vi "Save Image.vi"() -> ()   [LabVIEW 2013]
doc: "This VI imlements the framework and scheduler for your robotics program. It should not be necessary to modify the framework. You are expected to add your code to the VIs called from Robot Main, the ones located in the Team Code within the project."
panel:
  in  "Filename":string="Example.jpg"
  in  "Directory to save images":path=path "c:/images"
  out "Camera error":errorcluster
  out "File error":errorcluster
  out "Image":T1(plugin-control)
  in  "stop":bool
  in  "Save Image":bool
  # "This can be set\nwhile running."
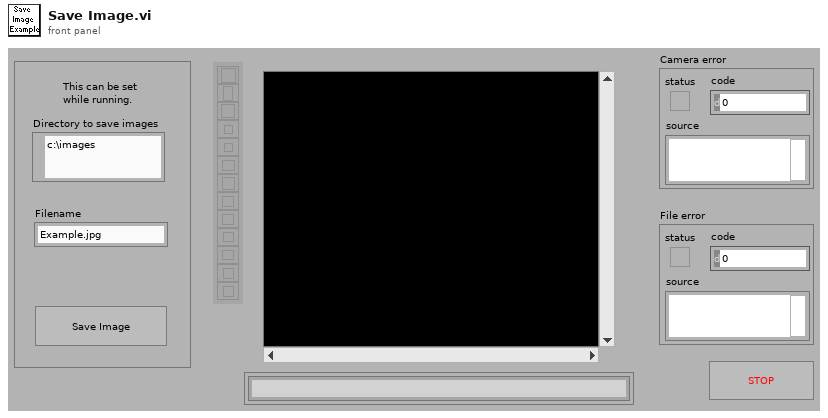
[diagram p1: front panel]
types:
  T1 = typedef "IMAQ Image.ctl" = refnum<image>
  T2 = typedef "Image Type" = u32
  T3 = typedef "WPI_CameraDevRef.ctl" = cluster{"Camera Address":string, "CameraStatus":errorcluster, "Acquire Image Notifier":refnum<notifier>}
  T4 = enum16{"open", "replace", "create", "open or create", "replace or create", "replace or create with confirmation"}
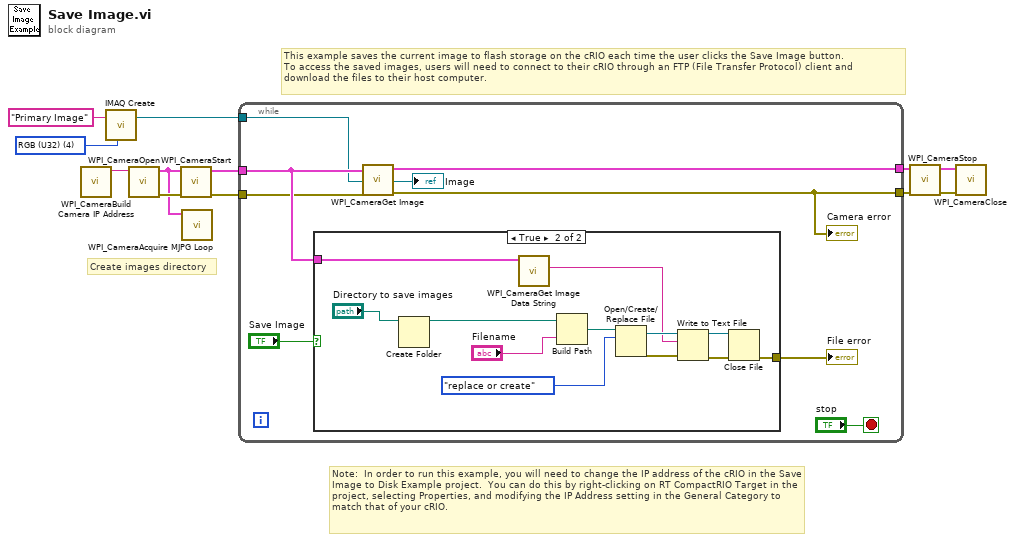
[diagram p0: block diagram]
diagram:
  w5 = T2 4 items=["Grayscale (U8)", "Grayscale (I16)", "Grayscale (SGL)", "Complex (CSG)", "RGB (U32)", "HSL (U32)", "RGB (U64)"] ("Image Type")
  # "Note:  In order to run this example, you will need to change the IP address of the cRIO in the Save Image to Disk Example project.  You can do this by right-clicking on RT CompactRIO Target in the project, selecting Properties, and modifying the IP Address setting in the General Category to match that of your cRIO."
  # "This example saves the current image to flash storage on the cRIO each time the user clicks the Save Image button.\nTo access the saved images, users will need to connect to their cRIO through an FTP (File Transfer Protocol) client and\ndownload the files to their host computer."
  # "Create images directory"
  n1 = call <vilib>:"WPI_CameraBuild Camera IP Address.vi"() -> ("Camera Address"=w1:string)  [unwired: 11 in]
  n2 = call "IMAQ Create"("Image Name"="Primary Image", "Image Type"=w5) -> ("New Image"=w3:T1)  [unwired: 2 in, 2 out]
  n3 = call <vilib>:"WPI_CameraOpen.vi"("Camera Address"=w1) -> ("error out"=w9:errorcluster, "CameraDevRef"=w2:T3)  [unwired: 1 in, 8 out]
  n4 = call <vilib>:"WPI_CameraStart.vi"("error in (no error)"=w9, "CameraDevRef"=w2) -> ("error out"=w8:errorcluster, "CameraDevRef Out"=w12:T3)  [unwired: 8 out]
  n5 = call <vilib>:"WPI_CameraAcquire MJPG Loop.vi"("CameraDevRef"=w2) -> ()  [unwired: 11 in]
  n6 = while {
    tunnel: w12 -> [w20]
    tunnel: [w19] -> w10
    tunnel: w8 -> [w17]
    tunnel: [w16] -> w7
    tunnel: w3 -> [w15]
    stop <- "stop" stop-if-true
    n7 = case shown="True" "Save Image" {
      tunnel: w20 -> [_ w28]
      tunnel: [_ w26] -> w13
      frame False {
      }
      frame True {
        n8 = Create Folder(path (use dialog)="Directory to save images") -> (created path=w22:path)  [unwired: 1 in, 3 out]
        n9 = call <vilib>:"WPI_CameraGet Image Data String.vi"("CameraDevRef"=w28) -> ("Image Data String"=w27:string)  [unwired: 1 in, 9 out]
        n10 = Build Path(base path=w22, name or relative path="Filename") -> (appended path=w25:path)
        n11 = Open/Create/Replace File(file path (use dialog)=w25, operation (0:open)=T4."replace or create") -> (refnum out=w31:refnum<file>, error out=w30:errorcluster)  [unwired: 1 in, 4 out]
        n12 = Write to Text File(file (use dialog)=w31, text=w27, error in=w30) -> (refnum out=w32:refnum<file>, error out=w29:errorcluster)  [unwired: 2 out]
        n13 = Close File(refnum=w32, error in=w29) -> (error out=w26:errorcluster)  [unwired: 1 out]
      }
    }
    "File error" <- w13
    n14 = call <vilib>:"WPI_CameraGet Image.vi"("error in (no error)"=w17, "Image"=w15, "CameraDevRef"=w20) -> ("error out"=w16:errorcluster, "Image Out"=→"Image":T1, "CameraDevRef Out"=w19:T3)  [unwired: 6 out]
    "Camera error" <- w16
  }
  n15 = call <vilib>:"WPI_CameraStop.vi"("error in (no error)"=w7, "CameraDevRef"=w10) -> ("error out"=w6:errorcluster, "CameraDevRef Out"=w11:T3)  [unwired: 8 out]
  n16 = call <vilib>:"WPI_CameraClose.vi"("error in (no error)"=w6, "CameraDevRef"=w11) -> ()  [unwired: 10 out]
